vi "kickfirstforce.vi"(6 "Target":dbl[](array[numeric]), 8 "error in (no error)":errorcluster, 9 "Robot":refnum<class "Robot.lvclass">, 10 "Game":refnum<class "Game.lvclass">, 11 "KickToSkill in":refnum<class "KickToSkill.lvclass">) -> (0 "error out":errorcluster, 1 "Orientation":dbl, 2 "Force":dbl, 3 "KickToSkill out":refnum<class "KickToSkill.lvclass">)   [LabVIEW 2023, in "KickToSkill.lvclass"]
uses:
  KickToSkill.lvclass
  Game_class/Game.lvclass
  Robot_class/Robot.lvclass
  C:/Users/ebert/Desktop/roboime/SSL_AI/Object_class/Object.lvclass
  Game_class/KickValueTest/Kickmeanvalues.ctl
  Game_class/Game.lvclass/Game.ctl
  Object_class/Object.lvclass/Object.ctl
  Ball_class/Ball.lvclass/Ball.ctl
  <vilib>/Analysis/coordinate.llb/2D Cartesian Coordinate Rotation (Scalar).vi
  Object_class/Read position(x,y).vi
  Game_class/Read BallRef.vi
  Ball_class/Read v_x.vi
  Ball_class/Read v_y.vi
  Ball_class/Ball.lvclass
  <vilib>/Analysis/NI_AALPro.lvlib
  Utilities_class/Utilities.lvclass
panel:
  in  "Teste":bool
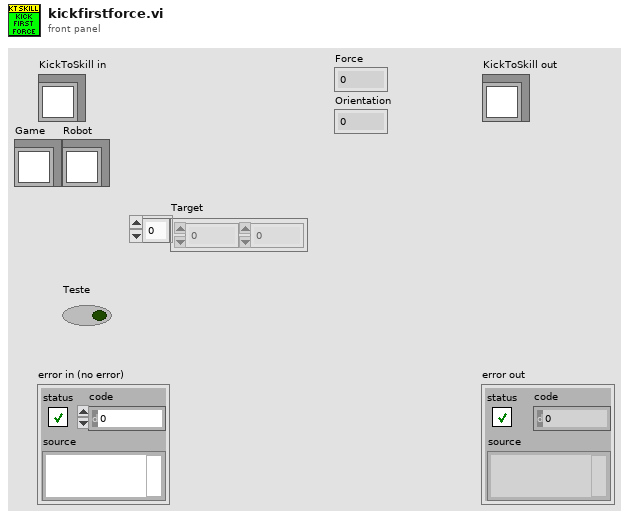
[diagram p1: front panel]
types:
  T1 = typedef "Kickmeanvalues.ctl" = dbl[][]
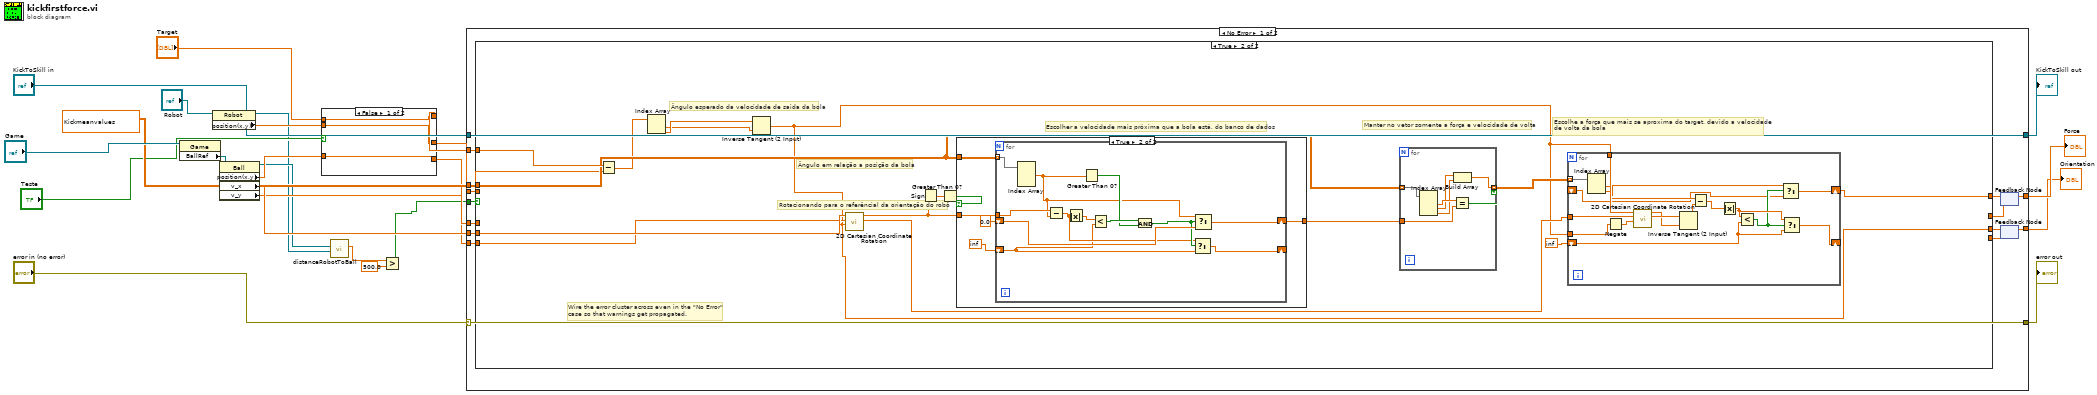
[diagram p0: block diagram]
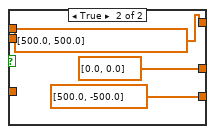
[diagram p2: hidden frame]
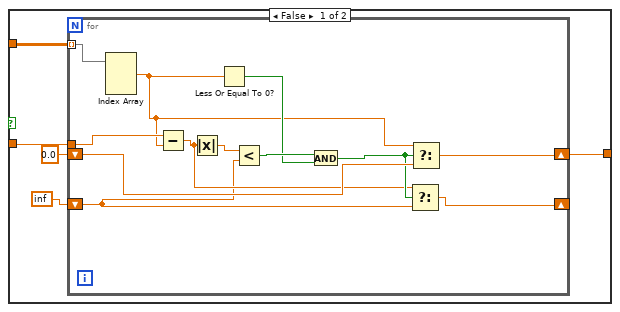
[diagram p4: hidden frame]
diagram:
  n1 = property class="Game"(reference="Game") -> ("BallRef"=w15:refnum<class "Ball.lvclass">)  [unwired: 1 in, 2 out]
  n2 = property class="Robot"(reference="Robot") -> (reference out=w4:refnum<class "Robot.lvclass">, "position(x,y)"=w10:dbl[])  [unwired: 1 in, 1 out]
  n3 = property class="Ball"(reference=w15) -> (reference out=w5:refnum<class "Ball.lvclass">, "position(x,y)"=w9:dbl[], "v_x"=w7:dbl, "v_y"=w6:dbl)  [unwired: 1 in, 1 out]
  n4 = case shown="False" "Teste" {
    tunnel: [w26 dbl[] [0.0, 0.0] ("position(x,y)")] -> w14
    tunnel: [w27 dbl[] [500.0, 500.0] ("Target")] -> w13
    tunnel: [w25 dbl[] [500.0, -500.0] ("position(x,y)")] -> w12
    tunnel: "Target" -> [w27 _]
    tunnel: w10 -> [w26 _]
    tunnel: w9 -> [w25 _]
    frame False {
    }
    frame True {
    }
  }
  n5 = call "distanceRobotToBall.vi"("Robot"=w4, "Ball"=w5) -> ("Distance Robot To Ball"=w3:dbl)  [unwired: 7 in, 2 out]
  n6 = Greater?(x=w3, y=500.0) -> (0:w1:bool)
  n7 = case shown="No Error" "error in (no error)" {
    selector: "error in (no error)" -> [w42 w122]
    tunnel: [w42 w122] -> w23
    tunnel: [w43 w121] -> w21
    tunnel: "KickToSkill in" -> [w43 w121]
    tunnel: w13 -> [w41 _]
    tunnel: T1 [[-4.0, 50.0, 3.274877129436019], [-4.0, 60.0, 4.143627251185135], [-4.0, 70.0, 2.701105442430398], [-4.0, 80.0, 2.899398392263049], [-4.0, 90.0, 2.7566434755503764], [-4.0, 100.0, 3.1909487542919313], [-3.0, 50.0, 3.3639282862390965], [-3.0, 60.0, 2.9052336433966133], [-3.0, 70.0, 3.3737278949344987], [-3.0, 80.0, 3.4555239478161606], [-3.0, 90.0, 3.4188584213607798], [-3.0, 100.0, 3.29704648585375], [-2.0, 50.0, 3.4168797011695435], [-2.0, 60.0, 3.5979584363670813], [-2.0, 70.0, 3.5810410501053007], [-2.0, 80.0, 3.3547691269742943], [-2.0, 90.0, 3.368842331838431], [-2.0, 100.0, 3.3547302687019798], [-1.0, 50.0, 3.3574503477639617], [-1.0, 60.0, 3.3417640159826627], [-1.0, 70.0, 3.04407567449978], [-1.0, 80.0, 3.2440153199141566], [-1.0, 90.0, 3.2448856638354098], [-1.0, 100.0, 3.3577211349914475], [0.0, 50.0, 3.3567610711849043], [0.0, 60.0, 3.3393019070216976], [0.0, 70.0, 3.354224093929638], [0.0, 80.0, 3.3697374962268167], [0.0, 90.0, 3.4324429478474396], [0.0, 100.0, 3.3490341749415196], [1.0, 50.0, 3.513340784643937], [1.0, 60.0, 3.46354055180706], [1.0, 70.0, 3.4204188556468975], [1.0, 80.0, 3.593593696187893], [1.0, 90.0, 3.54274876582048], [1.0, 100.0, 3.4868431049619075], [2.0, 50.0, 3.5850540313691437], [2.0, 60.0, 3.5291864149970777], [2.0, 70.0, 3.669538222219838], [2.0, 80.0, 3.5181089591372543], [2.0, 90.0, 3.6555360201674154], [2.0, 100.0, 3.651149714664325]] ("KickForceMean") -> [w40 _]
    tunnel: [w33 _] -> w18
    tunnel: [w31 _] -> w17
    tunnel: w14 -> [w39 _]
    tunnel: w12 -> [w36 _]
    tunnel: w7 -> [w38 _]
    tunnel: w6 -> [w37 _]
    tunnel: w1 -> [w35 _]
    frame No Error {
      n8 = feedback #1() -> (w31:dbl)  [unwired: 1 in]
      n9 = feedback #2() -> (w33:dbl)  [unwired: 1 in]
      n10 = case shown="True" w35 {
        tunnel: w41 -> [_ w62]
        tunnel: w40 -> [_ w57]
        tunnel: [w45 w53] -> w34
        tunnel: w39 -> [_ w52]
        tunnel: w38 -> [_ w51]
        tunnel: w37 -> [_ w50]
        tunnel: w36 -> [_ _]
        tunnel: [w44 w48] -> w32
        tunnel: w33 -> [w45 _]
        tunnel: w31 -> [w44 _]
        frame False {
        }
        frame True {
          # "Ângulo em relação a posição da bola"
          # "Ângulo esperado da velocidade de saida da bola"
          # "Escolhe a força que mais se aproxima do target, devido a velocidade\nde volta da bola"
          # "Manter no vetor somente a força e velocidade de volta"
          # "Escolher a velocidade mais próxima que a bola está, do banco de dados"
          # "Rotacionando para o referêncial da orientação do robô"
          # "Wire the error cluster across even in the \"No Error\"\ncase so that warnings get propagated."
          n11 = Subtract(x=w62, y=w52) -> (x-y=w49:dbl[])
          n12 = Index Array(array=w49) -> (element #1=w46:dbl, element #2=w47:dbl)  [unwired: 2 in]
          n13 = Inverse Tangent (2 Input)(1:w46, 2:w47) -> (0:w48:dbl)
          n14 = call-poly <vilib>:"2D Cartesian Coordinate Rotation.vi"("theta"=w48, "y"=w50, "x"=w51) -> ("y out"=w55:dbl, "x out"=w61:dbl)  [unwired: 6 in, 1 out]
          n15 = Sign(1:w61) -> (0:w60:dbl)
          n16 = Greater Than 0?(x=w60) -> (x > 0?=w59:bool)
          n17 = case shown="True" w59 {
            tunnel: w57 -> [w91 w108]
            tunnel: w61 -> [w90 w107]
            tunnel: [w89 w105] -> w58
            frame False {
              n18 = for {
                tunnel: w91 -> [w103] mode=indexing
                tunnel: w90 -> [w102]
                shift-right: [w94] -> _
                shift-left: inf -> [w92]
                shift-right: [w97] -> w89
                shift-left: 0.0 ("mean") -> [w96]
                n19 = Index Array(array=w103) -> (element #1=w98:dbl)  [unwired: 3 in, 2 out]
                n20 = Subtract(x=w102, y=w98) -> (x-y=w93:dbl)
                n21 = Absolute Value(x=w93) -> (abs(x)=w101:dbl)
                n22 = Less Or Equal To 0?(x=w98) -> (x <= 0?=w99:bool)
                n23 = Less?(x=w101, y=w92) -> (x < y?=w100:bool)
                n24 = And(x=w100, y=w99) -> (x .and. y?=w95:bool)
                n25 = Select(t=w93, s=w95, f=w92) -> (s? t:f=w94:dbl)
                n26 = Select(t=w98, s=w95, f=w96) -> (s? t:f=w97:dbl)
              }
            }
            frame True {
              n27 = for {
                tunnel: w108 -> [w120] mode=indexing
                tunnel: w107 -> [w119]
                shift-right: [w111] -> _
                shift-left: inf -> [w109]
                shift-right: [w114] -> w105
                shift-left: 0.0 ("mean") -> [w113]
                n28 = Index Array(array=w120) -> (element #1=w115:dbl)  [unwired: 3 in, 2 out]
                n29 = Subtract(x=w119, y=w115) -> (x-y=w110:dbl)
                n30 = Absolute Value(x=w110) -> (abs(x)=w118:dbl)
                n31 = Greater Than 0?(x=w115) -> (x > 0?=w116:bool)
                n32 = Less?(x=w118, y=w109) -> (x < y?=w117:bool)
                n33 = And(x=w117, y=w116) -> (x .and. y?=w112:bool)
                n34 = Select(t=w110, s=w112, f=w109) -> (s? t:f=w111:dbl)
                n35 = Select(t=w115, s=w112, f=w113) -> (s? t:f=w114:dbl)
              }
            }
          }
          n36 = for {
            tunnel: w58 -> [w84]
            tunnel: w57 -> [w86] mode=indexing
            tunnel: [w80] -> w56 mode=indexing if=w83
            n37 = Index Array(array=w86) -> (element #1=w85:dbl, element #2=w82:dbl, element #3=w81:dbl)  [unwired: 3 in]
            n38 = Build Array(w82, w81) -> (w80:dbl[])
            n39 = Equal?(x=w85, y=w84) -> (x = y?=w83:bool)
          }
          n40 = for {
            tunnel: w56 -> [w79] mode=indexing
            tunnel: w55 -> [w78]
            tunnel: w48 -> [w75]
            tunnel: w48 -> [w71]
            shift-right: [w68] -> _
            shift-left: inf -> [w69]
            shift-right: [w64] -> w53
            shift-left: _ -> [w63]
            n41 = Index Array(array=w79) -> (element #1=w65:dbl, element #2=w77:dbl)  [unwired: 2 in]
            n42 = Negate(x=w75) -> (-x=w76:dbl)
            n43 = call-poly <vilib>:"2D Cartesian Coordinate Rotation.vi"("theta"=w76, "y"=w78, "x"=w77) -> ("y out"=w74:dbl, "x out"=w73:dbl)  [unwired: 6 in, 1 out]
            n44 = Inverse Tangent (2 Input)(1:w73, 2:w74) -> (0:w72:dbl)
            n45 = Subtract(x=w71, y=w72) -> (x-y=w70:dbl)
            n46 = Absolute Value(x=w70) -> (abs(x)=w67:dbl)
            n47 = Less?(x=w67, y=w69) -> (x < y?=w66:bool)
            n48 = Select(t=w65, s=w66, f=w63) -> (s? t:f=w64:dbl)
            n49 = Select(t=w67, s=w66, f=w69) -> (s? t:f=w68:dbl)
          }
        }
      }
      n50 = feedback-in #1(w32) -> ()
      n51 = feedback-in #2(w34) -> ()
    }
    frame Error {
    }
  }
  "error out" <- w23
  "KickToSkill out" <- w21
  "Force" <- w18
  "Orientation" <- w17
